vi "run.vi"   [LabVIEW 2016, in "WRO2016.lvrbt"]
uses:
  WRO2016.lvrbt
  <vilib>/NXT/Block Support/NXT_InputPort.ctl
  <vilib>/NXT/Subs/ColorSensorColors.ctl
  <vilib>/NXT/Hardware/Plugins/Tetrix DC Motor/TetrixDCMotorAddress.ctl
  <vilib>/NXT/Hardware/Plugins/Tetrix 180 deg Servo/Tetrix180ServoAddress.ctl
  <vilib>/NXT/NXTIO Xnodes/NXTIONodeSubVIs/TETRIX IO Move Servos.vi
  <vilib>/NXT/Dual Mode Library/Waits/Wait_Num.vi
  <vilib>/NXT/NXTIO Xnodes/NXTIONodeSubVIs/TETRIX IO Move DC Motors.vi
  <vilib>/NXT/NXTIO Xnodes/NXTIONodeSubVIs/TETRIX IO Stop DC Motors.vi
  <vilib>/NXT/Dual Mode Library/Waits/Wait_EV3_Ultrasonic_Centimeter_Closer.vi
  <vilib>/NXT/Dual Mode Library/Waits/Wait_EV3_Ultrasonic_Centimeters_Further.vi
  <vilib>/NXT/Dual Mode Library/Waits/Wait_EV3_Color_Color.vi
  <vilib>/NXT/NXTIO Xnodes/AddressXNode/NXTIOAddress.xnode
  <vilib>/NXT/Subs/LVHSConnector.ctl
  <vilib>/NXT/NXTIO Xnodes/NXTIOXNode/NXTIO.xnode
  <vilib>/NXT/LegoClasses/BrickReference/BrickReference.lvclass
types:
  T1 = typedef "NXT_InputPort.ctl" = u32
  T2 = typedef "ColorSensorColors.ctl" = enum16{"No Color", "Black", "Blue", "Green", "Yellow", "Red", "White", "Brown"}
  T3 = typedef "Tetrix180ServoAddress.ctl" = i32
  T4 = cluster{"Tetrix180Servo":T3, "Tetrix180Servo":T3, "Tetrix180Servo":T3, "Tetrix180Servo":T3, "Tetrix180Servo":T3}
  T5 = typedef "LVHSConnector.ctl" = refnum<class "BrickReference.lvclass">
  T6 = typedef "TetrixDCMotorAddress.ctl" = i32
diagram:
  w3 = T1 1 items=["Port 1", "Port 2", "Port 3", "Port 4"] ("Port (Port 1)")
  w157 = T1 1 items=["Port 1", "Port 2", "Port 3", "Port 4"] ("Port (Port 1)")
  w171 = T1 1 items=["Port 1", "Port 2", "Port 3", "Port 4"] ("Port (Port 1)")
  w179 = T1 1 items=["Port 1", "Port 2", "Port 3", "Port 4"] ("Port (Port 1)")
  w180 = T1 1 items=["Port 1", "Port 2", "Port 3", "Port 4"] ("Port (Port 1)")
  # "Function 3:\n\nThe servo is prepared to grab the ball"
  # "Function 7:\n\nReady  to go back to base."
  # "Function 6:\nRelease the first ball."
  # "Function 5 (c):\n\nPrepare for the aim position"
  # "REMIND TO CHECK BEFORE RUNNNING!!!"
  # "Function 5 (b):\n\nThe servo will put the ball into the servo 4"
  # "Function 5 (a):\n\nThe ball is ready to get the aim"
  # "Function 4:\n\nTher servo motor will lock the ball"
  # "REMIND TO CHECK BEFORE RUNNNING!!!"
  # "REMIND TO CHECK BEFORE RUNNNING!!!"
  # "REMIND TO CHECK BEFORE RUNNNING!!!"
  # "Function 2 (b):\n\nThe robot is getting the position to take the ball inside the rack."
  # "Function 2(a):\n\nThe robot will start to detect the rack with the ultra sonic sensor."
  # "Function 1:\n\nOut from the based to start the game."
  n1 = xnode "Motors"() -> ("Motor"=w206:T4)
  n2 = xnode "Move Servos"("Position 5"=u8 0, "Position 4"=u8 40, "Position 3"=u8 0, "Position 2"=u8 0, "Position 1"=u8 255, "Motors"=w206) -> ("NXT/EV3"=w199:T5)  [unwired: 1 in]
  n3 = xnode "Motors"() -> ("Motor"=w209:cluster{"TetrixDCMotor":T6, "TetrixDCMotor":T6})
  n4 = call-poly <vilib>:"PolyWait.vi"("Time (1 sec)"=sgl 1.0, "NXT/EV3"=w199) -> ("NXT/EV3"=w198:T5)  [unwired: 2 in]
  n5 = xnode "Move Motors"("Power/Speed 1"=i8 100, "Motors"=w209, "NXT/EV3"=w198, "Power/Speed 2"=i8 100) -> ("NXT/EV3"=w214:T5)
  n6 = call-poly <vilib>:"PolyWait.vi"("Time (1 sec)"=sgl 2.0, "NXT/EV3"=w214) -> ("NXT/EV3"=w210:T5)  [unwired: 2 in]
  n7 = xnode "Stop Motors"("Motors"=w209, "NXT/EV3"=w210) -> ("NXT/EV3"=w207:T5)
  n8 = xnode "Motors"() -> ("Motor"=w192:cluster{"TetrixDCMotor":T6, "TetrixDCMotor":T6})
  n9 = call-poly <vilib>:"PolyWait.vi"("Time (1 sec)"=sgl 1.0, "NXT/EV3"=w207) -> ("NXT/EV3"=w161:T5)  [unwired: 2 in]
  n10 = xnode "Move Motors"("Power/Speed 2"=i8 100, "Power/Speed 1"=i8 100, "Motors"=w192, "NXT/EV3"=w161) -> ("NXT/EV3"=w195:T5)
  n11 = call-poly <vilib>:"PolyWait.vi"("Centimeters (40)"=sgl 6.5, "NXT/EV3"=w195, "Port (Port 1)"=w180) -> ("NXT/EV3"=w193:T5)  [unwired: 1 in]
  n12 = xnode "Stop Motors"("Motors"=w192, "NXT/EV3"=w193) -> ("NXT/EV3"=w191:T5)
  n13 = xnode "Motors"() -> ("Motor"=w183:cluster{"TetrixDCMotor":T6, "TetrixDCMotor":T6})
  n14 = call-poly <vilib>:"PolyWait.vi"("Time (1 sec)"=sgl 1.0, "NXT/EV3"=w191) -> ("NXT/EV3"=w189:T5)  [unwired: 2 in]
  n15 = xnode "Move Motors"("Power/Speed 2"=i8 20, "Power/Speed 1"=i8 21, "Motors"=w183, "NXT/EV3"=w189) -> ("NXT/EV3"=w186:T5)
  n16 = call-poly <vilib>:"PolyWait.vi"("Centimeters (50)"=sgl 5.0, "NXT/EV3"=w186, "Port (Port 1)"=w179) -> ("NXT/EV3"=w184:T5)  [unwired: 1 in]
  n17 = xnode "Stop Motors"("Motors"=w183, "NXT/EV3"=w184) -> ("NXT/EV3"=w181:T5)
  n18 = xnode "Motors"() -> ("Motor"=w174:cluster{"TetrixDCMotor":T6, "TetrixDCMotor":T6})
  n19 = call-poly <vilib>:"PolyWait.vi"("Time (1 sec)"=sgl 1.0, "NXT/EV3"=w181) -> ("NXT/EV3"=w172:T5)  [unwired: 2 in]
  n20 = xnode "Move Motors"("Power/Speed 2"=i8 -5, "Power/Speed 1"=i8 -5, "Motors"=w174, "NXT/EV3"=w172) -> ("NXT/EV3"=w176:T5)
  n21 = call-poly <vilib>:"PolyWait.vi"("Centimeters (40)"=sgl 5.0, "NXT/EV3"=w176, "Port (Port 1)"=w171) -> ("NXT/EV3"=w175:T5)  [unwired: 1 in]
  n22 = xnode "Stop Motors"("Motors"=w174, "NXT/EV3"=w175) -> ("NXT/EV3"=w166:T5)
  n23 = xnode "Motors"() -> ("Motor"=w163:cluster{"TetrixDCMotor":T6, "TetrixDCMotor":T6})
  n24 = call-poly <vilib>:"PolyWait.vi"("Time (1 sec)"=sgl 1.0, "NXT/EV3"=w166) -> ("NXT/EV3"=w167:T5)  [unwired: 2 in]
  n25 = xnode "Move Motors"("Power/Speed 2"=i8 5, "Power/Speed 1"=i8 5, "Motors"=w163, "NXT/EV3"=w167) -> ("NXT/EV3"=w164:T5)
  n26 = call-poly <vilib>:"PolyWait.vi"("Time (1 sec)"=sgl 0.6, "NXT/EV3"=w164) -> ("NXT/EV3"=w162:T5)  [unwired: 2 in]
  n27 = xnode "Stop Motors"("Motors"=w163, "NXT/EV3"=w162) -> ("NXT/EV3"=w131:T5)
  n28 = xnode "Motors"() -> ("Motor"=w152:T3)
  n29 = call-poly <vilib>:"PolyWait.vi"("Time (1 sec)"=sgl 1.0, "NXT/EV3"=w131) -> ("NXT/EV3"=w133:T5)  [unwired: 2 in]
  n30 = xnode "Move Servos"("Position 1"=u8 108, "Motors"=w152, "NXT/EV3"=w133) -> ("NXT/EV3"=w149:T5)
  n31 = call-poly <vilib>:"PolyWait.vi"("Time (1 sec)"=sgl 7.0, "NXT/EV3"=w149) -> ("NXT/EV3"=w146:T5)  [unwired: 2 in]
  n32 = xnode "Motors"() -> ("Motor"=w148:T3)
  n33 = xnode "Move Servos"("Position 1"=u8 227, "Motors"=w148, "NXT/EV3"=w146) -> ("NXT/EV3"=w144:T5)
  n34 = xnode "Motors"() -> ("Motor"=w143:T3)
  n35 = call-poly <vilib>:"PolyWait.vi"("Time (1 sec)"=sgl 0.5, "NXT/EV3"=w144) -> ("NXT/EV3"=w141:T5)  [unwired: 2 in]
  n36 = xnode "Move Servos"("Position 1"=u8 15, "Motors"=w143, "NXT/EV3"=w141) -> ("NXT/EV3"=w139:T5)
  n37 = call-poly <vilib>:"PolyWait.vi"("Time (1 sec)"=sgl 1.5, "NXT/EV3"=w139) -> ("NXT/EV3"=w136:T5)  [unwired: 2 in]
  n38 = xnode "Motors"() -> ("Motor"=w137:T3)
  n39 = xnode "Move Servos"("Position 1"=u8 98, "Motors"=w137, "NXT/EV3"=w136) -> ("NXT/EV3"=w135:T5)
  n40 = xnode "Motors"() -> ("Motor"=w155:cluster{"TetrixDCMotor":T6, "TetrixDCMotor":T6})
  n41 = call-poly <vilib>:"PolyWait.vi"("Time (1 sec)"=sgl 1.0, "NXT/EV3"=w135) -> ("NXT/EV3"=w153:T5)  [unwired: 2 in]
  n42 = xnode "Move Motors"("Power/Speed 2"=i8 5, "Power/Speed 1"=i8 5, "Motors"=w155, "NXT/EV3"=w153) -> ("NXT/EV3"=w158:T5)
  n43 = call-poly <vilib>:"PolyWait.vi"("Centimeters (50)"=sgl 5.0, "NXT/EV3"=w158, "Port (Port 1)"=w157) -> ("NXT/EV3"=w156:T5)  [unwired: 1 in]
  n44 = xnode "Stop Motors"("Motors"=w155, "NXT/EV3"=w156) -> ("NXT/EV3"=w119:T5)
  n45 = call-poly <vilib>:"PolyWait.vi"("Time (1 sec)"=sgl 1.0, "NXT/EV3"=w119) -> ("NXT/EV3"=w127:T5)  [unwired: 2 in]
  n46 = xnode "Motors"() -> ("Motor"=w128:T3)
  n47 = xnode "Move Servos"("Position 1"=u8 67, "Motors"=w128, "NXT/EV3"=w127) -> ("NXT/EV3"=w125:T5)
  n48 = call-poly <vilib>:"PolyWait.vi"("Time (1 sec)"=sgl 1.0, "NXT/EV3"=w125) -> ("NXT/EV3"=w122:T5)  [unwired: 2 in]
  n49 = xnode "Motors"() -> ("Motor"=w123:T3)
  n50 = xnode "Move Servos"("Position 1"=u8 240, "Motors"=w123, "NXT/EV3"=w122) -> ("NXT/EV3"=w120:T5)
  n51 = xnode "Motors"() -> ("Motor"=w113:cluster{"TetrixDCMotor":T6, "TetrixDCMotor":T6})
  n52 = call-poly <vilib>:"PolyWait.vi"("Time (1 sec)"=sgl 1.0, "NXT/EV3"=w120) -> ("NXT/EV3"=w103:T5)  [unwired: 2 in]
  n53 = xnode "Move Motors"("Power/Speed 2"=i8 -100, "Power/Speed 1"=i8 -100, "Motors"=w113, "NXT/EV3"=w103) -> ("NXT/EV3"=w115:T5)
  n54 = call-poly <vilib>:"PolyWait.vi"("Time (1 sec)"=sgl 1.0, "NXT/EV3"=w115) -> ("NXT/EV3"=w114:T5)  [unwired: 2 in]
  n55 = xnode "Stop Motors"("Motors"=w113, "NXT/EV3"=w114) -> ("NXT/EV3"=w111:T5)
  n56 = xnode "Motors"() -> ("Motor"=w104:cluster{"TetrixDCMotor":T6, "TetrixDCMotor":T6})
  n57 = call-poly <vilib>:"PolyWait.vi"("Time (1 sec)"=sgl 1.0, "NXT/EV3"=w111) -> ("NXT/EV3"=w108:T5)  [unwired: 2 in]
  n58 = xnode "Move Motors"("Power/Speed 2"=i8 -100, "Power/Speed 1"=i8 -100, "Motors"=w104, "NXT/EV3"=w108) -> ("NXT/EV3"=w106:T5)
  n59 = call-poly <vilib>:"PolyWait.vi"("Time (1 sec)"=sgl 1.0, "NXT/EV3"=w106) -> ("NXT/EV3"=w105:T5)  [unwired: 2 in]
  n60 = xnode "Stop Motors"("Motors"=w104, "NXT/EV3"=w105) -> ("NXT/EV3"=w88:T5)
  n61 = call-poly <vilib>:"PolyWait.vi"("Time (1 sec)"=sgl 1.0, "NXT/EV3"=w88) -> ("NXT/EV3"=w99:T5)  [unwired: 2 in]
  n62 = xnode "Motors"() -> ("Motor"=w100:T3)
  n63 = xnode "Move Servos"("Position 1"=u8 0, "Motors"=w100, "NXT/EV3"=w99) -> ("NXT/EV3"=w97:T5)
  n64 = xnode "Motors"() -> ("Motor"=w95:T3)
  n65 = call-poly <vilib>:"PolyWait.vi"("Time (1 sec)"=sgl 1.0, "NXT/EV3"=w97) -> ("NXT/EV3"=w94:T5)  [unwired: 2 in]
  n66 = xnode "Move Servos"("Position 1"=u8 255, "Motors"=w95, "NXT/EV3"=w94) -> ("NXT/EV3"=w92:T5)
  n67 = call-poly <vilib>:"PolyWait.vi"("Time (1 sec)"=sgl 1.0, "NXT/EV3"=w92) -> ("NXT/EV3"=w89:T5)  [unwired: 2 in]
  n68 = xnode "Motors"() -> ("Motor"=w90:T3)
  n69 = xnode "Move Servos"("Position 1"=u8 0, "Motors"=w90, "NXT/EV3"=w89) -> ("NXT/EV3"=w77:T5)
  n70 = xnode "Motors"() -> ("Motor"=w80:cluster{"TetrixDCMotor":T6, "TetrixDCMotor":T6})
  n71 = call-poly <vilib>:"PolyWait.vi"("Time (1 sec)"=sgl 1.5, "NXT/EV3"=w77) -> ("NXT/EV3"=w86:T5)  [unwired: 2 in]
  n72 = xnode "Move Motors"("Power/Speed 2"=i8 10, "Power/Speed 1"=i8 10, "Motors"=w80, "NXT/EV3"=w86) -> ("NXT/EV3"=w83:T5)
  n73 = xnode "Motors"() -> ("Sensor"=w5:T1)
  n74 = call-poly <vilib>:"PolyWait.vi"("Color (Red)"=ColorSensorColors."Black", "NXT/EV3"=w83, "Port (Port 1)"=w5) -> ("NXT/EV3"=w81:T5)  [unwired: 1 in]
  n75 = xnode "Stop Motors"("Motors"=w80, "NXT/EV3"=w81) -> ("NXT/EV3"=w78:T5)
  n76 = call-poly <vilib>:"PolyWait.vi"("Time (1 sec)"=sgl 1.5, "NXT/EV3"=w78) -> ("NXT/EV3"=w76:T5)  [unwired: 2 in]
  n77 = xnode "Motors"() -> ("Motor"=w75:T3)
  n78 = xnode "Move Servos"("Position 1"=u8 118, "Motors"=w75, "NXT/EV3"=w76) -> ("NXT/EV3"=w72:T5)
  n79 = call-poly <vilib>:"PolyWait.vi"("Time (1 sec)"=sgl 1.5, "NXT/EV3"=w72) -> ("NXT/EV3"=w69:T5)  [unwired: 2 in]
  n80 = xnode "Motors"() -> ("Motor"=w71:T3)
  n81 = xnode "Move Servos"("Position 1"=u8 40, "Motors"=w71, "NXT/EV3"=w69) -> ("NXT/EV3"=w61:T5)
  n82 = xnode "Motors"() -> ("Motor"=w63:cluster{"TetrixDCMotor":T6, "TetrixDCMotor":T6})
  n83 = call-poly <vilib>:"PolyWait.vi"("Time (1 sec)"=sgl 2.0, "NXT/EV3"=w61) -> ("NXT/EV3"=w60:T5)  [unwired: 2 in]
  n84 = xnode "Move Motors"("Power/Speed 2"=i8 -75, "Power/Speed 1"=i8 -75, "Motors"=w63, "NXT/EV3"=w60) -> ("NXT/EV3"=w66:T5)
  n85 = xnode "Motors"() -> ("Sensor"=w4:T1)
  n86 = call-poly <vilib>:"PolyWait.vi"("Color (Red)"=ColorSensorColors."Black", "NXT/EV3"=w66, "Port (Port 1)"=w4) -> ("NXT/EV3"=w64:T5)  [unwired: 1 in]
  n87 = xnode "Stop Motors"("Motors"=w63, "NXT/EV3"=w64) -> ("NXT/EV3"=w8:T5)
  n88 = call-poly <vilib>:"PolyWait.vi"("Time (1 sec)"=sgl 1.0, "NXT/EV3"=w8) -> ("NXT/EV3"=w56:T5)  [unwired: 2 in]
  n89 = xnode "Motors"() -> ("Motor"=w7:cluster{"TetrixDCMotor":T6, "TetrixDCMotor":T6})
  n90 = xnode "Move Motors"("Power/Speed 2"=i8 -10, "Power/Speed 1"=i8 -10, "Motors"=w7, "NXT/EV3"=w56) -> ("NXT/EV3"=w54:T5)
  n91 = call-poly <vilib>:"PolyWait.vi"("Centimeters (40)"=sgl 4.5 ("Time (1 sec)"), "NXT/EV3"=w54, "Port (Port 1)"=w3) -> ("NXT/EV3"=w53:T5)  [unwired: 1 in]
  n92 = xnode "Stop Motors"("Motors"=w7, "NXT/EV3"=w53) -> ("NXT/EV3"=w36:T5)
  n93 = xnode "Motors"() -> ("Motor"=w42:cluster{"TetrixDCMotor":T6, "TetrixDCMotor":T6})
  n94 = call-poly <vilib>:"PolyWait.vi"("Time (1 sec)"=sgl 1.0, "NXT/EV3"=w36) -> ("NXT/EV3"=w41:T5)  [unwired: 2 in]
  n95 = xnode "Move Motors"("Power/Speed 2"=i8 -75, "Power/Speed 1"=i8 -75, "Motors"=w42, "NXT/EV3"=w41) -> ("NXT/EV3"=w43:T5)
  n96 = call-poly <vilib>:"PolyWait.vi"("Time (1 sec)"=sgl 0.2, "NXT/EV3"=w43) -> ("NXT/EV3"=w44:T5)  [unwired: 2 in]
  n97 = xnode "Stop Motors"("Motors"=w42, "NXT/EV3"=w44) -> ("NXT/EV3"=w38:T5)
  n98 = call-poly <vilib>:"PolyWait.vi"("Time (1 sec)"=sgl 0.5, "NXT/EV3"=w38) -> ("NXT/EV3"=w37:T5)  [unwired: 2 in]
  n99 = xnode "Motors"() -> ("Motor"=w6:cluster{"TetrixDCMotor":T6, "TetrixDCMotor":T6})
  n100 = xnode "Move Motors"("Power/Speed 2"=i8 -75, "Power/Speed 1"=i8 -75, "Motors"=w6, "NXT/EV3"=w37) -> ("NXT/EV3"=w47:T5)
  n101 = xnode "Motors"() -> ("Sensor"=w2:T1)
  n102 = call-poly <vilib>:"PolyWait.vi"("Color (Red)"=ColorSensorColors."Black", "NXT/EV3"=w47, "Port (Port 1)"=w2) -> ("NXT/EV3"=w48:T5)  [unwired: 1 in]
  n103 = xnode "Stop Motors"("Motors"=w6, "NXT/EV3"=w48) -> ("NXT/EV3"=w16:T5)
  n104 = xnode "Motors"() -> ("Motor"=w30:cluster{"TetrixDCMotor":T6, "TetrixDCMotor":T6})
  n105 = call-poly <vilib>:"PolyWait.vi"("Time (1 sec)"=sgl 0.5, "NXT/EV3"=w16) -> ("NXT/EV3"=w19:T5)  [unwired: 2 in]
  n106 = xnode "Move Motors"("Power/Speed 2"=i8 75, "Power/Speed 1"=i8 75, "Motors"=w30, "NXT/EV3"=w19) -> ("NXT/EV3"=w31:T5)
  n107 = xnode "Motors"() -> ("Sensor"=w1:T1)
  n108 = call-poly <vilib>:"PolyWait.vi"("Color (Red)"=ColorSensorColors."Black", "NXT/EV3"=w31, "Port (Port 1)"=w1) -> ("NXT/EV3"=w32:T5)  [unwired: 1 in]
  n109 = xnode "Stop Motors"("Motors"=w30, "NXT/EV3"=w32) -> ("NXT/EV3"=w28:T5)
  n110 = xnode "Motors"() -> ("Motor"=w21:cluster{"TetrixDCMotor":T6, "TetrixDCMotor":T6})
  n111 = call-poly <vilib>:"PolyWait.vi"("Time (1 sec)"=sgl 1.0, "NXT/EV3"=w28) -> ("NXT/EV3"=w25:T5)  [unwired: 2 in]
  n112 = xnode "Move Motors"("Power/Speed 2"=i8 -75, "Power/Speed 1"=i8 -75, "Motors"=w21, "NXT/EV3"=w25) -> ("NXT/EV3"=w23:T5)
  n113 = call-poly <vilib>:"PolyWait.vi"("Time (1 sec)"=sgl 0.85, "NXT/EV3"=w23) -> ("NXT/EV3"=w22:T5)  [unwired: 2 in]
  n114 = xnode "Stop Motors"("Motors"=w21, "NXT/EV3"=w22) -> ("NXT/EV3"=w18:T5)
  n115 = call-poly <vilib>:"PolyWait.vi"("Time (1 sec)"=sgl 1.0, "NXT/EV3"=w18) -> ("NXT/EV3"=w9:T5)  [unwired: 2 in]
  n116 = xnode "Motors"() -> ("Motor"=w15:T4)
  n117 = xnode "Move Servos"("Position 5"=u8 200, "Position 4"=u8 40, "Position 3"=u8 0, "Position 2"=u8 0, "Position 1"=u8 255, "Motors"=w15, "NXT/EV3"=w9) -> ()  [unwired: 1 out]
